vi "Connection Mode Generation Queue Messages.vi"(0 "J1939 Cluster":T7, 5 "Connection Refs":T1, 11 "error in":errorcluster) -> (13 "Message Error":errorcluster, 15 "System Error out":errorcluster)   [LabVIEW 2015, in "J1939 Addon Engine.lvlib"]
uses:
  J1939 Addon Engine.lvlib
  Types/Setup Information Cluster.ctl
  <vilib>/xnet/xnet.llb/XNET Frame CAN.ctl
  <vilib>/xnet/xnet.llb/XNET Frame Type CAN.ctl
  Shared/J1939 Utilities/Types/CAN Outgoing Message Cluster.ctl
  Types/TP List References.ctl
  Types/BAM Buffer Connections List_Ref.ctl
  Types/TP Buffer Connection Cluster.ctl
  Types/Connection Mode Generation Connection Ref.ctl
  Types/Connection Mode Generation Connection Cluster.ctl
  Types/BAM Generation Connections List_Ref.ctl
  Types/BAM Generation Connection Cluster.ctl
  Types/Address Table Reference.ctl
  Types/RQST Lookup Table Reference.ctl
  Types/TP Connections List State.ctl
  Connection Mode Generation Connections List_Actions.vi
  Connection Mode Generation Get Next Messages.vi
  Shared/J1939 Utilities/SubVIs/TP.Conn Abort.vi
  Shared/J1939 Utilities/Common Conversions.vi
  Shared/J1939 Utilities/SubVIs/Convert J1939 ID to CAN Arb ID.vi
  Connection Mode Generation Connections List.vi
  Shared/J1939 Utilities/J1939 Utilities.lvlib
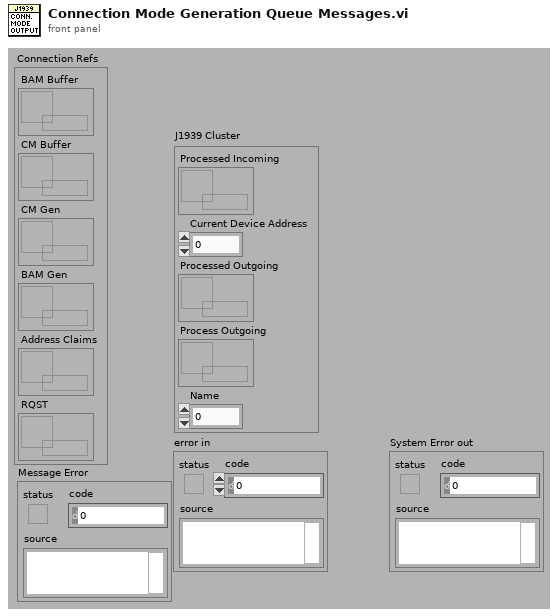
[diagram p1: front panel]
types:
  T1 = typedef "J1939 Addon Engine.lvlib/TP List References.ctl" = cluster{"BAM Buffer":T2, "CM Buffer":T2, "CM Gen":T3, "BAM Gen":T4, "Address Claims":T5, "RQST":T6}
  T2 = typedef "J1939 Addon Engine.lvlib/BAM Buffer Connections List_Ref.ctl" = refnum<data-value>
  T3 = typedef "J1939 Addon Engine.lvlib/Connection Mode Generation Connection Ref.ctl" = refnum<data-value>
  T4 = typedef "J1939 Addon Engine.lvlib/BAM Generation Connections List_Ref.ctl" = refnum<data-value>
  T5 = typedef "J1939 Addon Engine.lvlib/Address Table Reference.ctl" = refnum<data-value>
  T6 = typedef "J1939 Addon Engine.lvlib/RQST Lookup Table Reference.ctl" = refnum<data-value>
  T7 = typedef "J1939 Addon Engine.lvlib/Setup Information Cluster.ctl" = cluster{"Processed Incoming":refnum<queue>, "Current Device Address":u8, "Processed Outgoing":refnum<queue>, "Process Outgoing":refnum<queue>, "Name":u64}
  T8 = typedef "J1939 Addon Engine.lvlib/TP Connections List State.ctl" = enum16{"Add", "Update", "Get", "Remove", "Initialize"}
  T9 = typedef "J1939 Addon Engine.lvlib/Connection Mode Generation Connection Cluster.ctl" = cluster{"Total Packets":u8, "Current Packet to Generate":u8, "Packets":T10[], "Previous Time Stamp":u32, "Total Bytes":u16, "Packet Identifier [PDU S + SA]":u16, "Number of Packets to Generate":u8, "PGN":u32}
  T10 = typedef "J1939 Addon Shared.lvlib/J1939 Utilities.lvlib/CAN Outgoing Message Cluster.ctl" = cluster{"Identifier":u32, "Data":u8[]}
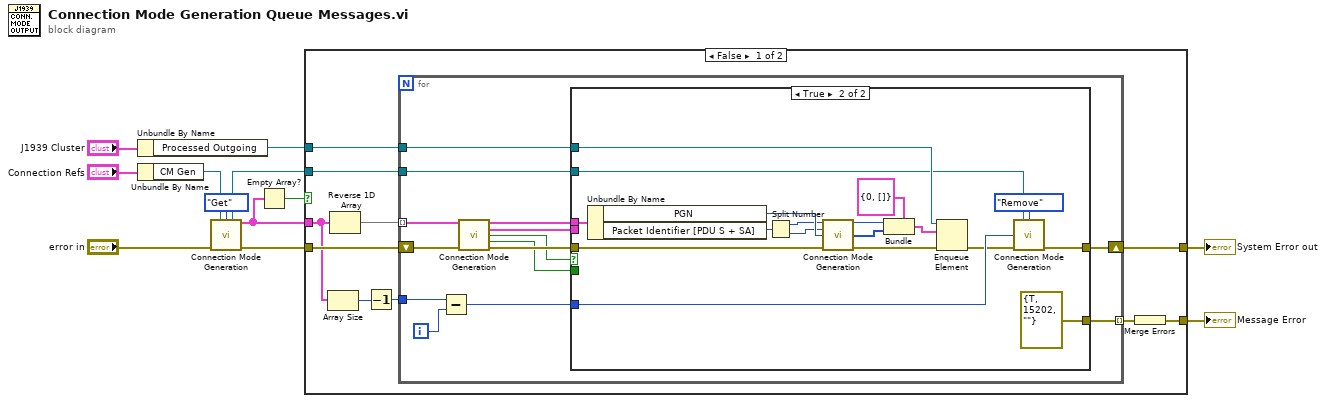
[diagram p0: block diagram]
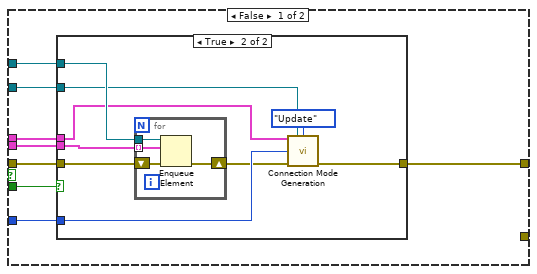
[diagram p2: hidden frame]
diagram:
  n1 = Unbundle By Name("J1939 Cluster") -> ("Processed Outgoing"=w5:refnum<queue>)
  n2 = Unbundle By Name("Connection Refs") -> ("CM Gen"=w3:T3)
  n3 = call-poly "Connection Mode Generation.vi"("CM Gen Ref"=w3, "State"=TP_Connections_List_State."Get", "error in (no error)"="error in") -> ("CM Gen Ref out"=w2:T3, "Connections"=w11:T9[], "error out"=w10:errorcluster)  [unwired: 2 in, 8 out]
  n4 = Empty Array?(array=w11) -> (empty?=w9:bool)
  n5 = case shown="False" w9 {
    tunnel: w10 -> [w22 w77]
    tunnel: w11 -> [w20 _]
    tunnel: w5 -> [w17 _]
    tunnel: [w16 w77] -> w12
    tunnel: w2 -> [w15 _]
    tunnel: [w13 _] -> w1
    frame False {
      n6 = Array Size(array=w20) -> (size(s)=w19:i32)
      n7 = Reverse 1D Array(array=w20) -> (reversed array=w21:T9[])
      n8 = Decrement(x=w19) -> (x-1=w18:i32)
      n9 = for {
        tunnel: w21 -> [w35] mode=indexing
        tunnel: w18 -> [w32]
        shift-right: [w29] -> w16
        shift-left: w22 -> [w36]
        tunnel: w17 -> [w26]
        tunnel: w15 -> [w24]
        tunnel: [w23] -> w14 mode=indexing
        i -> [w31]
        n10 = Subtract(x=w32, y=w31) -> (x-y=w30:i32)
        n11 = call-poly "Connection Mode Generation.vi"("Connection Cluster"=w35, "error in (no error)"=w36) -> ("Connection Cluster"=w33:T9, "Data to Send Array"=w25:T10[], "Timeout?"=w28:bool, "Message Available?"=w27:bool, "error out"=w34:errorcluster)  [unwired: 9 out]
        n12 = case shown="True" w28 {
          tunnel: w34 -> [w44 w76]
          tunnel: w33 -> [w43 w75]
          tunnel: w30 -> [w42 w70]
          tunnel: [w41 w68] -> w29
          tunnel: w27 -> [w40 _]
          tunnel: w26 -> [w39 w62]
          tunnel: w25 -> [w38 _]
          tunnel: w24 -> [w37 w60]
          tunnel: [_ errorcluster {"status"=TRUE, "code"=15202, "source"=""} ("error out")] -> w23
          frame False {
            n13 = case shown="True" w40 {
              tunnel: w44 -> [w45 w51]
              tunnel: w43 -> [_ w48]
              tunnel: w42 -> [_ w53]
              tunnel: [w45 w52] -> w41
              tunnel: w39 -> [_ w49]
              tunnel: w38 -> [_ w47]
              tunnel: w37 -> [_ w46]
              frame False {
              }
              frame True {
                n14 = for {
                  tunnel: w49 -> [w56]
                  tunnel: w47 -> [w55] mode=indexing
                  shift-right: [w57] -> w50
                  shift-left: w51 -> [w58]
                  n15 = Enqueue Element(queue=w56, element=w55, error in (no error)=w58) -> (error out=w57:errorcluster)  [unwired: 3 out]
                }
                n16 = call-poly "Connection Mode Generation.vi"("Connection Cluster"=w48, "CM Gen Ref"=w46, "State"=TP_Connections_List_State."Update", "index"=w53, "error in (no error)"=w50) -> ("error out"=w52:errorcluster)  [unwired: 10 out]
              }
            }
          }
          frame True {
            n17 = Unbundle By Name(w75) -> ("PGN"=w74:u32, "Packet Identifier [PDU S + SA]"=w73:u16)
            n18 = Split Number(x=w73) -> (hi(x)=w72:u8, lo(x)=w71:u8)
            n19 = call-poly "Connection Mode Generation.vi"("Destination Address"=w72, "Source Address"=w71, "PGN"=w74, "error in (no error)"=w76) -> ("Arb ID"=w65:u32, "Data"=w64:u8[], "error out"=w67:errorcluster)  [unwired: 9 out]
            n20 = Bundle(cluster=T10 {"Identifier"=0, "Data"=[]} ("Data to Send"), "Identifier"=w65, "Data"=w64) -> (w63:T10)
            n21 = Enqueue Element(queue=w62, element=w63, error in (no error)=w67) -> (error out=w66:errorcluster)  [unwired: 3 out]
            n22 = call-poly "Connection Mode Generation.vi"("CM Gen Ref"=w60, "State"=TP_Connections_List_State."Remove", "index"=w70, "error in (no error)"=w66) -> ("error out"=w68:errorcluster)  [unwired: 1 in, 10 out]
          }
        }
      }
      n23 = Merge Errors(w14) -> (w13:errorcluster)
    }
    frame True {
    }
  }
  "System Error out" <- w12
  "Message Error" <- w1
